vi "Reset.vi"(8 "error in (no error)":errorcluster, 11 "VISA resource name":refnum<visa-resource-name>) -> (0 "error out":errorcluster, 3 "VISA resource name out":refnum<visa-resource-name>)   [LabVIEW 2010]
doc: "Resets the instrument and then sends a set of default setup commands to the instrument."
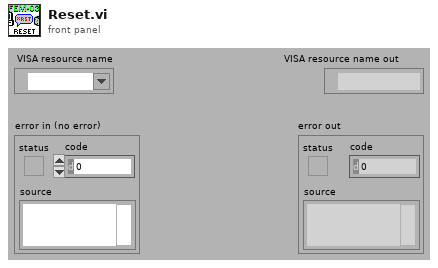
[diagram p1: front panel]
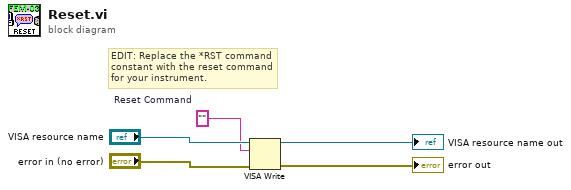
[diagram p0: block diagram]
diagram:
  w3 = ""  # Reset Command
  # "EDIT: Replace the *RST command\nconstant with the reset command\nfor your instrument."
  n1 = VISA Write(VISA resource name="VISA resource name", write buffer=w3, error in (no error)="error in (no error)") -> (VISA resource name out=→"VISA resource name out":refnum<visa-resource-name>, error out=→"error out":errorcluster)  [unwired: 1 out]
